vi "3D(SubVI).vi"(6 "Y array":dbl[](array[numeric]), 9 "X array":dbl[](array[numeric]), 10 "Array in":u32[](array[numeric]), 11 "altitude (cm)":u32) -> (2 "3D Graph":refnum<class "Base Datatype.lvclass">[](xcontrol), 3 "Array out":u32[](array[numeric]))   [LabVIEW 2014]
uses:
  <vilib>/Native 3D Graph/xcontrol/3DPC_SurfacePlot.xctl
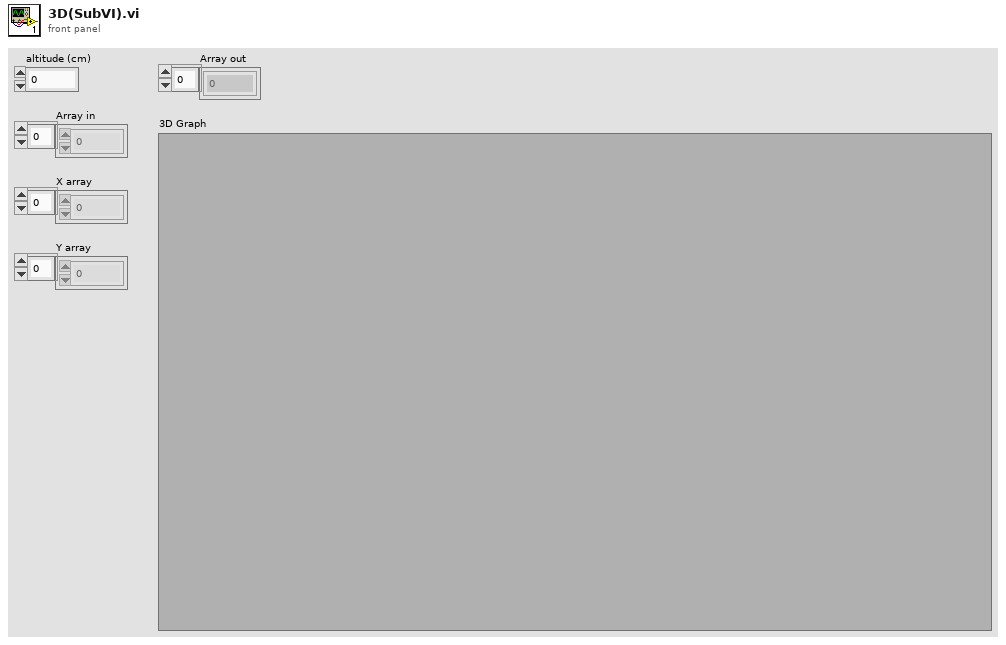
[diagram p1: front panel]
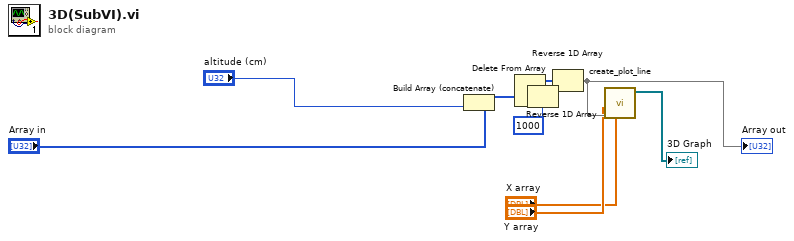
[diagram p0: block diagram]
diagram:
  n1 = Build Array (concatenate)("Array in", "altitude (cm)") -> (w4:u32[])
  n2 = Reverse 1D Array(array=w4) -> (reversed array=w5:u32[])
  n3 = Delete From Array(array=w5, index=1000) -> (array with subset deleted=w6:u32[])  [unwired: 1 in, 1 out]
  n4 = Reverse 1D Array(array=w6) -> (reversed array=w8:u32[])
  "Array out" <- w8
  n5 = call <vilib>:"create_plot_line.vi"("z vector"=w8, "y vector"="Y array", "x vector"="X array") -> ("plots out"=→"3D Graph":refnum<class "Base Datatype.lvclass">[])  [unwired: 2 in, 6 out]
